vi "LabView.vi"() -> ()   [LabVIEW 2023]
panel:
  in  "Output Ampefier":dbl
  in  "Out Of Bounds Level":dbl
  in  "Tolerance Level":dbl
  out "Out of Bounds":bool
  in  "stop":bool
  out "Back Right":dbl(knob) scale=-100.0..100.0
  out "Back Left":dbl(knob) scale=-100.0..100.0
  out "Front Right":dbl(knob) scale=-100.0..100.0
  out "Front Left":dbl(knob) scale=-100.0..100.0
  in  "RightLeft/Y rotation":dbl
  in  "FrontBack/X rotation":dbl
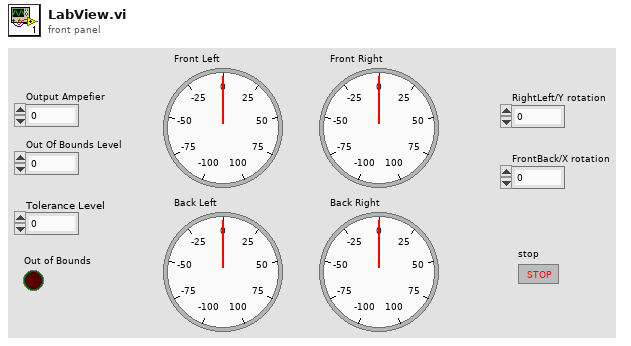
[diagram p1: front panel]
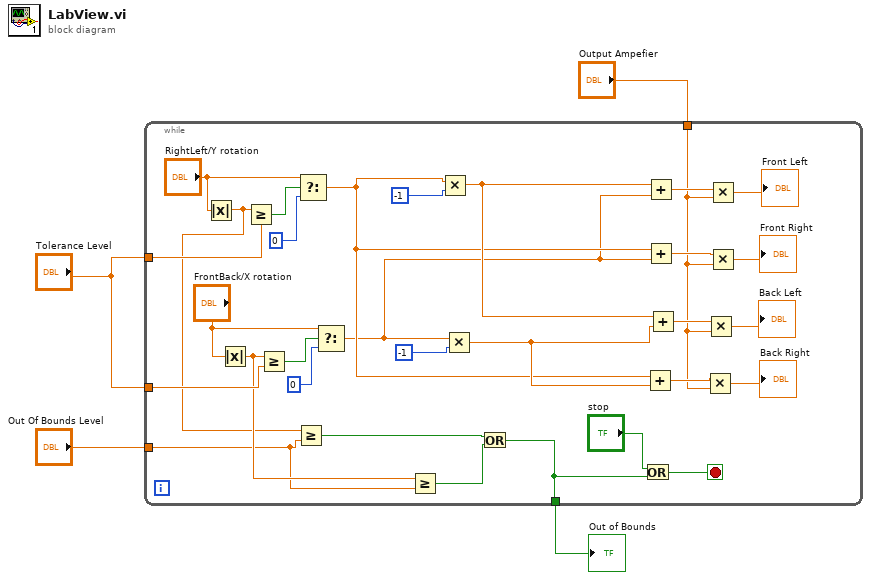
[diagram p0: block diagram]
diagram:
  n1 = while {
    tunnel: "Tolerance Level" -> [w28]
    tunnel: "Tolerance Level" -> [w23]
    tunnel: "Out Of Bounds Level" -> [w15]
    tunnel: [w14] -> w2
    tunnel: "Output Ampefier" -> [w9]
    stop <- w19 stop-if-true
    n2 = Absolute Value(x="RightLeft/Y rotation") -> (abs(x)=w16:dbl)
    n3 = Absolute Value(x="FrontBack/X rotation") -> (abs(x)=w17:dbl)
    n4 = Greater Or Equal?(x=w16, y=w28) -> (x >= y?=w27:bool)
    n5 = Greater Or Equal?(x=w17, y=w23) -> (x >= y?=w26:bool)
    n6 = Greater Or Equal?(x=w16, y=w15) -> (x >= y?=w21:bool)
    n7 = Select(t="RightLeft/Y rotation", s=w27, f=0) -> (s? t:f=w31:dbl)
    n8 = Select(t="FrontBack/X rotation", s=w26, f=0) -> (s? t:f=w24:dbl)
    n9 = Greater Or Equal?(x=w17, y=w15) -> (x >= y?=w20:bool)
    n10 = Multiply(x=w31, y=-1) -> (x*y=w32:dbl)
    n11 = Multiply(x=w24, y=-1) -> (x*y=w33:dbl)
    n12 = Or(x=w21, y=w20) -> (x .or. y?=w14:bool)
    n13 = Or(x="stop", y=w14) -> (x .or. y?=w19:bool)
    n14 = Add(x=w31, y=w33) -> (x+y=w13:dbl)
    n15 = Add(x=w32, y=w24) -> (x+y=w10:dbl)
    n16 = Add(x=w31, y=w24) -> (x+y=w11:dbl)
    n17 = Add(x=w32, y=w33) -> (x+y=w12:dbl)
    n18 = Multiply(x=w13, y=w9) -> (x*y=→"Back Right":dbl)
    n19 = Multiply(x=w12, y=w9) -> (x*y=→"Back Left":dbl)
    n20 = Multiply(x=w10, y=w9) -> (x*y=→"Front Left":dbl)
    n21 = Multiply(x=w11, y=w9) -> (x*y=→"Front Right":dbl)
  }
  "Out of Bounds" <- w2
